vi "Piccolo Decode Raw Data.vi"(8 "error in (no error)":errorcluster, 11 "U32 Array":u32[](array[numeric]) format="%05x") -> (0 "error out":errorcluster, 1 "Y array":u8[](array[numeric]), 2 "X array":u8[](array[numeric]), 3 "TDC Bins":u16[](array[numeric]), 4 "Event Info":u32[](array[numeric]))   [LabVIEW 2021, in "Piccolo.lvlib"]
uses:
  Piccolo.lvlib
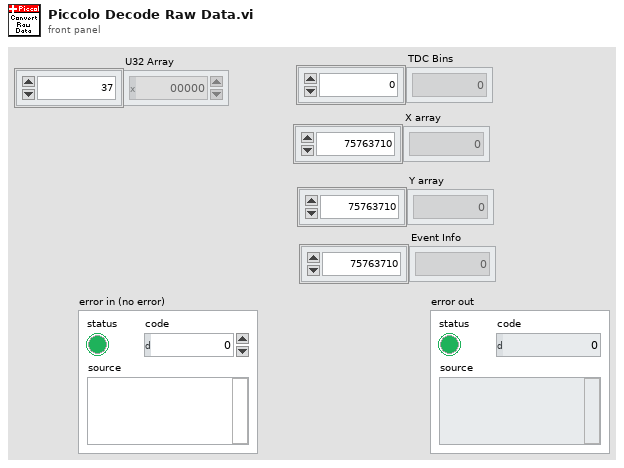
[diagram p1: front panel]
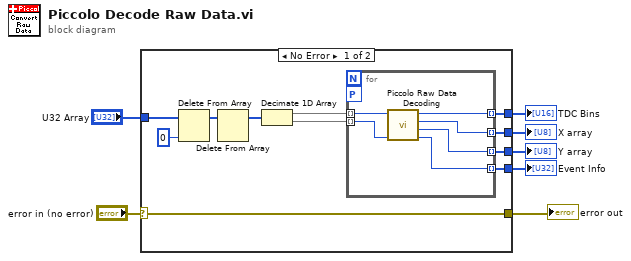
[diagram p0: block diagram]
diagram:
  n1 = case shown="No Error" "error in (no error)" {
    selector: "error in (no error)" -> [w8 w25]
    tunnel: "U32 Array" -> [w18 _]
    tunnel: [w17 _] -> w6
    tunnel: [w11 _] -> w5
    tunnel: [w10 _] -> w4
    tunnel: [w9 _] -> w3
    tunnel: [w8 w25] -> w1
    frame No Error {
      n2 = Delete From Array(array=w18, index=0) -> (array with subset deleted=w16:u32[])  [unwired: 1 in, 1 out]
      n3 = Delete From Array(array=w16) -> (array with subset deleted=w15:u32[])  [unwired: 2 in, 1 out]
      n4 = Decimate 1D Array(w15) -> (w13:u32[], w12:u32[])
      n5 = for {
        tunnel: w13 -> [w24] mode=indexing
        workers-P: _ -> [_]
        tunnel: [w23] -> w17 mode=indexing
        tunnel: w12 -> [w22] mode=indexing
        tunnel: [w21] -> w11 mode=indexing
        tunnel: [w20] -> w10 mode=indexing
        tunnel: [w19] -> w9 mode=indexing
        n6 = call "Piccolo Raw Data Decoding.vi"("TDC U32"=w22, "Photon U32"=w24) -> ("TDC U32"=w19:u32, "Y"=w20:u8, "X"=w21:u8, "TDC Bin"=w23:u16)  [unwired: 6 in]
      }
    }
    frame Error {
    }
  }
  "error out" <- w1
  "TDC Bins" <- w6
  "X array" <- w5
  "Y array" <- w4
  "Event Info" <- w3
